vi "tearDown.vi"(8 "error in (no error)":errorcluster, 11 "reference in":refnum<class "Switch Consumer Test Case.lvclass">) -> (0 "error out":errorcluster, 3 "reference out":refnum<class "Switch Consumer Test Case.lvclass">)   [LabVIEW 2017, in "Switch Consumer Test Case.lvclass"]
doc: "tearDown runs after the test method has completed. Use this method to clean up any operations or references that were opened by setUp or the test method. Unit tests should be independent of other unit tests so this VI should ensure that the next test can run in a 'clean' test environment."
uses:
  Switch Consumer Test Case.lvclass
  Switch Consumer Test Case.lvclass/Switch Consumer Test Case.ctl
  Consumer/Abstract Consumer/Abstract Consumer.lvclass
  Producer/Abstract Producer/Abstract Producer.lvclass
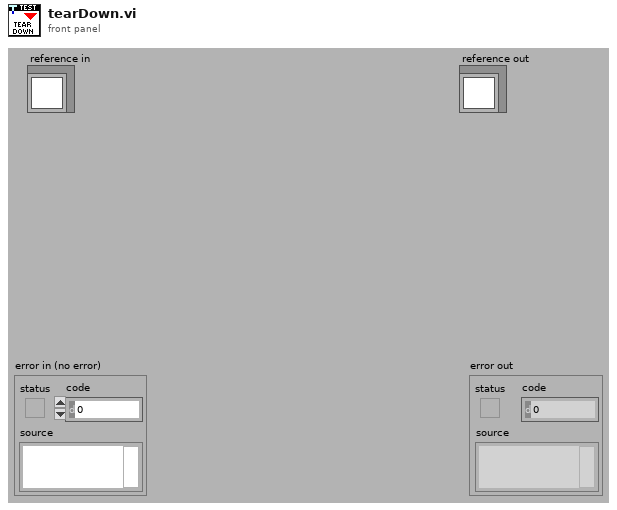
[diagram p1: front panel]
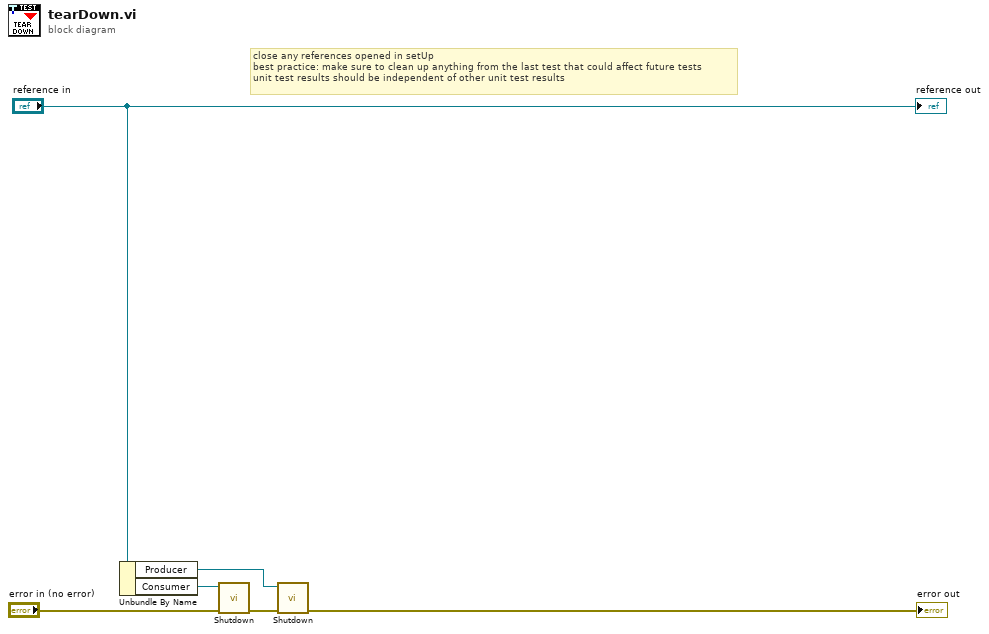
[diagram p0: block diagram]
diagram:
  # "close any references opened in setUp\nbest practice: make sure to clean up anything from the last test that could affect future tests\nunit test results should be independent of other unit test results"
  n1 = Unbundle By Name("reference in") -> ("Producer"=w1:refnum<class "Abstract Producer.lvclass">, "Consumer"=w5:refnum<class "Abstract Consumer.lvclass">)
  n2 = call "Shutdown.vi"("error in (no error)"="error in (no error)", "Abstract Consumer in"=w5) -> ("error out"=w3:errorcluster)  [unwired: 8 in, 1 out]
  n3 = call "Shutdown.vi"("error in (no error)"=w3, "Abstract Producer in"=w1) -> ("error out"=→"error out":errorcluster)  [unwired: 8 in, 1 out]
  "reference out" <- "reference in"
